vi "stringtotimestamp(sub).vi"(1 "string":string) -> (0 "Time Stamp":timestamp)   [LabVIEW 2015]
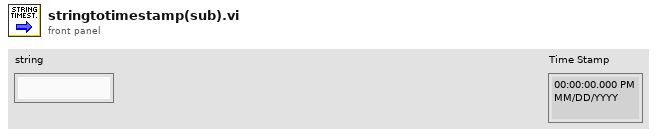
[diagram p1: front panel]
types:
  T1 = cluster{"second":i32, "minute":i32, "hour":i32, "day of month":i32, "month":i32, "year":i32, "day of week":i32, "day of year":i32, "is DST":i32}
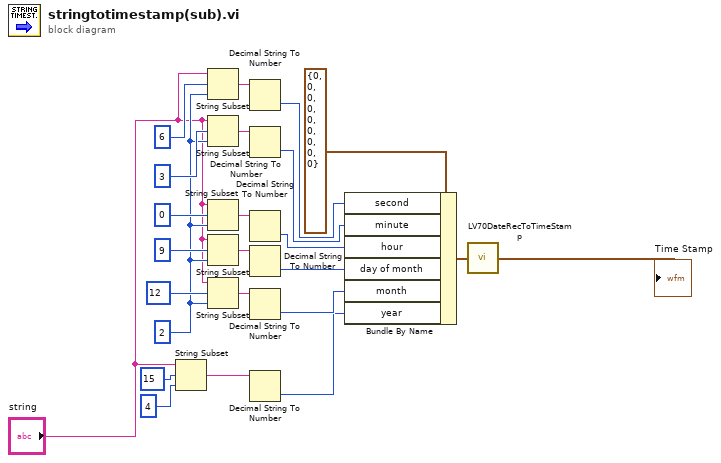
[diagram p0: block diagram]
diagram:
  w11 = 2 ("length (rest)")
  n1 = String Subset(string="string", offset (0)=15, length (rest)=4 ("length (rest)")) -> (substring=w13:string)
  n2 = String Subset(string="string", offset (0)=6, length (rest)=w11) -> (substring=w19:string)
  n3 = String Subset(string="string", offset (0)=3, length (rest)=w11) -> (substring=w21:string)
  n4 = String Subset(string="string", offset (0)=0, length (rest)=w11) -> (substring=w23:string)
  n5 = String Subset(string="string", offset (0)=9, length (rest)=w11) -> (substring=w17:string)
  n6 = String Subset(string="string", offset (0)=12, length (rest)=w11) -> (substring=w15:string)
  n7 = Decimal String To Number(string=w19) -> (number=w7:i32)  [unwired: 2 in, 1 out]
  n8 = Decimal String To Number(string=w21) -> (number=w5:i32)  [unwired: 2 in, 1 out]
  n9 = Decimal String To Number(string=w23) -> (number=w6:i32)  [unwired: 2 in, 1 out]
  n10 = Decimal String To Number(string=w17) -> (number=w4:i32)  [unwired: 2 in, 1 out]
  n11 = Decimal String To Number(string=w15) -> (number=w3:i32)  [unwired: 2 in, 1 out]
  n12 = Decimal String To Number(string=w13) -> (number=w2:i32)  [unwired: 2 in, 1 out]
  n13 = Bundle By Name(cluster=T1 {"second"=0, "minute"=0, "hour"=0, "day of month"=0, "month"=0, "year"=0, "day of week"=0, "day of year"=0, "is DST"=0} ("date time rec"), "second"=w7, "minute"=w5, "hour"=w6, "day of month"=w4, "month"=w3, "year"=w2) -> (w9:T1)
  n14 = call <vilib>:"LV70DateRecToTimeStamp.vi"("date time rec"=w9) -> ("Time Stamp"=→"Time Stamp":timestamp)
